vi "New Prop C.vi"(11 "GIC Input":T1={"     Use ?\nOff       On"=[FALSE, TRUE, FALSE, TRUE], "Mode:"=FALSE, "WP Data"="", "Hokuyo Port"="COM7", "Prop  Port"="COM6", "Compass Port"="", "GPS Port"="", "Num of WPs"=0, "WP Lats and Longs"={"WP Lats"=[], "WP Longs"=[]}, "Obst Lats and Longs"={"Obst Lats"=[], "Obst Longs"=[]}, "Parameters"=[], "GPS Data"=[], "Compass"=0.0, "LMS Vector"=[], "Vision Vector"=[], "Direction Cmd"=0.0, "Speed Cmd"=0.0, "WP Vector"=[], "WP Number"=0, "Extra"=0, "SW Map"=[], "Path Cluster"={"Path x node"=[], "Path y node"=[]}} {"Obst Lats and Longs"."Obst Longs" format="%#_8g"; "Obst Lats and Longs"."Obst Lats" format="%#_8g"}) -> ()   [LabVIEW 2014]
uses:
  RLcmd Global.vi
  FRcmd Global.vi
  <vilib>/Instr/_visa.llb/VISA Configure Serial Port (Instr).vi
panel:
  out "Prop VISA Resource Name":refnum<visa-resource-name>
  # "New Prop C"
  # "Input:"
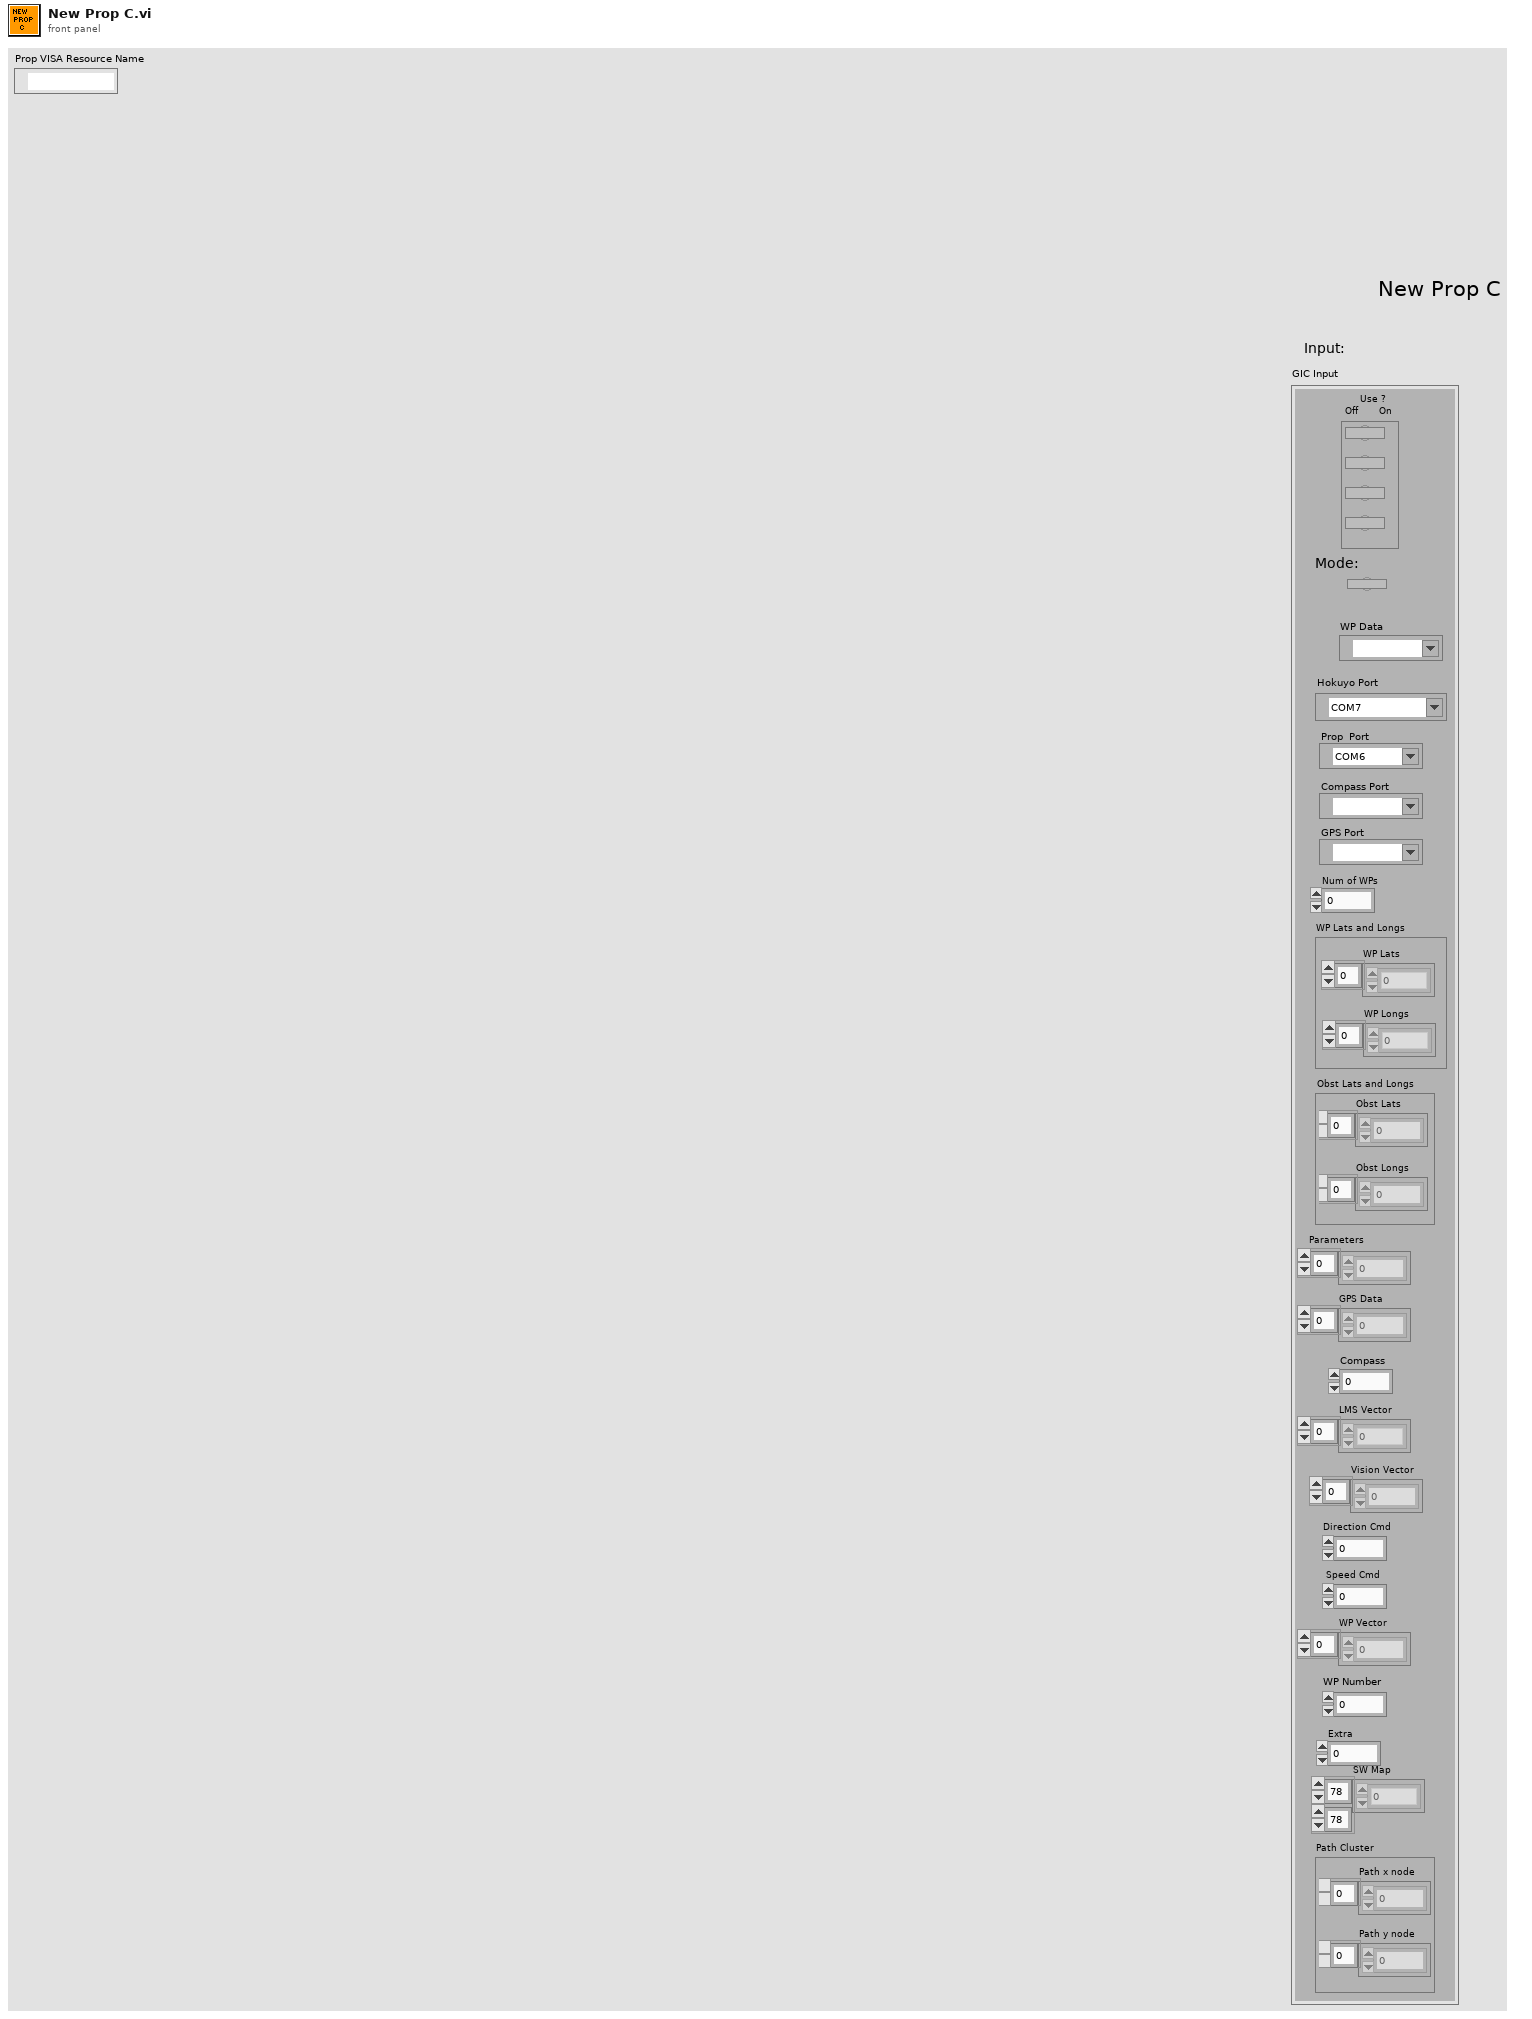
[diagram p1: front panel]
types:
  T1 = cluster{"     Use ?\nOff       On":bool[], "Mode:":bool, "WP Data":refnum<visa-resource-name>, "Hokuyo Port":refnum<visa-resource-name>, "Prop  Port":refnum<visa-resource-name>, "Compass Port":refnum<visa-resource-name>, "GPS Port":refnum<visa-resource-name>, "Num of WPs":i16, "WP Lats and Longs":cluster{"WP Lats":dbl[], "WP Longs":dbl[]}, "Obst Lats and Longs":cluster{"Obst Lats":dbl[], "Obst Longs":dbl[]}, "Parameters":dbl[], "GPS Data":dbl[], "Compass":dbl, "LMS Vector":dbl[], "Vision Vector":dbl[], "Direction Cmd":dbl, "Speed Cmd":dbl, "WP Vector":dbl[], "WP Number":i32, "Extra":i16, "SW Map":i32[][], "Path Cluster":cluster{"Path x node":dbl[], "Path y node":dbl[]}}
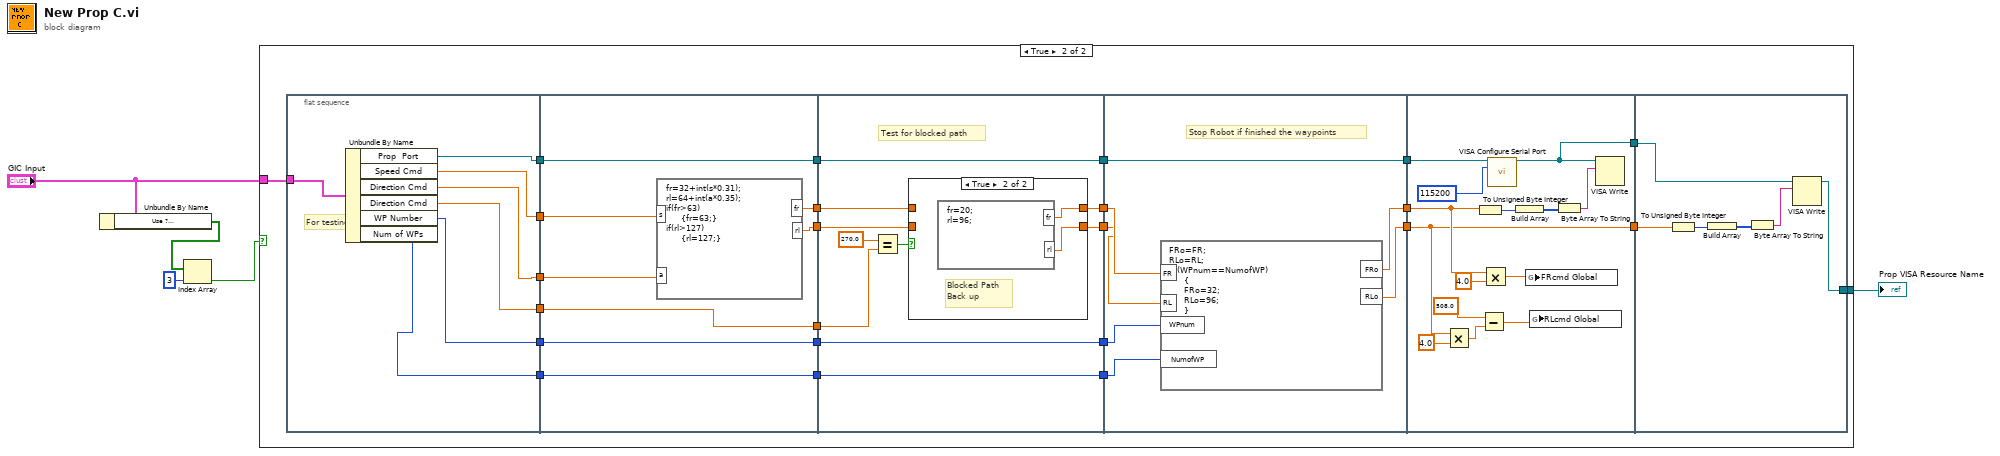
[diagram p0: block diagram]
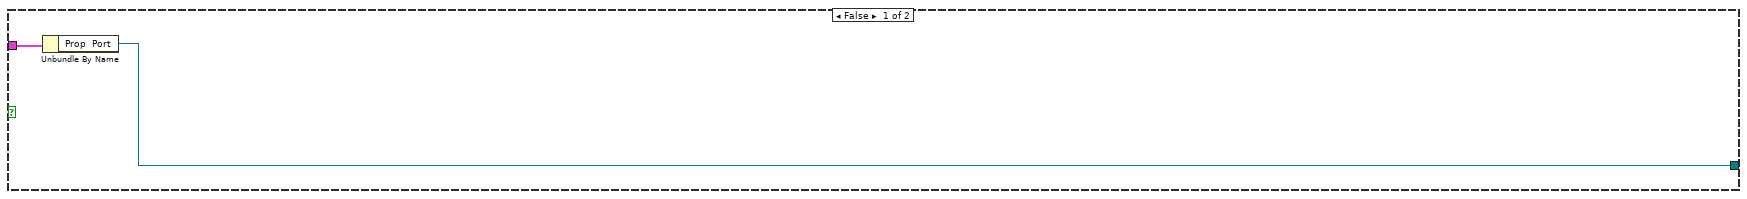
[diagram p2: hidden frame]
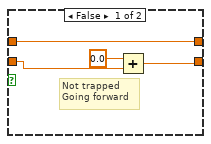
[diagram p3: hidden frame]
diagram:
  n1 = Unbundle By Name("GIC Input") -> ("Use ?\nOff       On"=w5:bool[])
  n2 = Index Array(array=w5, index=3) -> (element=w3:bool)
  n3 = case shown="True" w3 {
    tunnel: "GIC Input" -> [w7 w25]
    tunnel: [w6 w8] -> w2
    frame False {
      n4 = Unbundle By Name(w7) -> ("Prop  Port"=w6:refnum<visa-resource-name>)
    }
    frame True {
      n5 = flat-sequence {
        tunnel: [w38] -> w24
        tunnel: [w37] -> w23
        tunnel: [w36] -> w22
        tunnel: [w35] -> w21
        tunnel: w25 -> [w34]
        tunnel: [w33] -> w12
        tunnel: [w32] -> w9
        tunnel: [w46] -> w31
        tunnel: [w43] -> w30
        tunnel: [w42] -> w29
        tunnel: [w41] -> w28
        tunnel: w21 -> [w41]
        tunnel: w22 -> [w44]
        tunnel: w23 -> [w45]
        tunnel: w24 -> [w46]
        tunnel: [w40] -> w13
        tunnel: w12 -> [w40]
        tunnel: [w39] -> w10
        tunnel: w9 -> [w39]
        tunnel: w31 -> [w56]
        tunnel: [w56] -> w20
        tunnel: w30 -> [w52]
        tunnel: [w51] -> w18
        tunnel: w29 -> [w50]
        tunnel: [w49] -> w16
        tunnel: w28 -> [w53]
        tunnel: [w48] -> w14
        tunnel: w13 -> [w48]
        tunnel: [w47] -> w11
        tunnel: w10 -> [w47]
        tunnel: w20 -> [w69]
        tunnel: [w69] -> w19
        tunnel: w18 -> [w68]
        tunnel: [w66] -> w17
        tunnel: w16 -> [w67]
        tunnel: [w65] -> w15
        tunnel: w14 -> [w64]
        tunnel: w11 -> [w63]
        tunnel: [w79] -> w27
        tunnel: w19 -> [w78]
        tunnel: w17 -> [w77]
        tunnel: [w73] -> w26
        tunnel: w15 -> [w73]
        tunnel: w27 -> [w86]
        tunnel: w26 -> [w85]
        tunnel: [w84] -> w8
        frame #0 {
          # "For testing:"
          n6 = Unbundle By Name(w34) -> ("Prop  Port"=w38:refnum<visa-resource-name>, "Speed Cmd"=w37:dbl, "Direction Cmd"=w36:dbl, "Direction Cmd"=w35:dbl, "WP Number"=w33:i32, "Num of WPs"=w32:i16)
        }
        frame #1 {
          n7 = formula code="fr=32+int(s*0.31);\nrl=64+int(a*0.35);\nif(fr>63)\n     {fr=63;}\nif(rl>127)\n     {rl=127;}"("s"=w45, "a"=w44) -> ("fr"=w43:dbl, "rl"=w42:dbl)
        }
        frame #2 {
          # "Test for blocked path"
          n8 = Equal?(x=270.0, y=w53) -> (x = y?=w55:bool)
          n9 = case shown="True" w55 {
            tunnel: w52 -> [w60 _]
            tunnel: [w60 w62] -> w51
            tunnel: w50 -> [w58 _]
            tunnel: [w59 w61] -> w49
            frame False {
              # "Not trapped\nGoing forward"
              n10 = Add(x=0.0, y=w58) -> (x+y=w59:dbl)
            }
            frame True {
              # "Blocked Path\nBack up"
              n11 = formula code="fr=20;\nrl=96;"() -> ("fr"=w62:dbl, "rl"=w61:dbl)
            }
          }
        }
        frame #3 {
          # "Stop Robot if finished the waypoints"
          n12 = formula code="FRo=FR;\nRLo=RL;\nif (WPnum==NumofWP)\n     {\n     FRo=32;\n     RLo=96;\n     }"("FR"=w68, "RL"=w67, "WPnum"=w64, "NumofWP"=w63) -> ("FRo"=w66:dbl, "RLo"=w65:dbl)
        }
        frame #4 {
          n13 = Multiply(x=w73, y=4.0) -> (x*y=w71:dbl)
          n14 = To Unsigned Byte Integer(number=w77) -> (unsigned 8bit integer=w81:u8)
          n15 = Subtract(x=508.0, y=w71) -> (x-y=w70:dbl)
          n16 = Multiply(x=w77, y=4.0) -> (x*y=w75:dbl)
          n17 = call-poly "VISA Configure Serial Port"("VISA resource name"=w78, "baud rate (9600)"=115200) -> ("VISA resource name out"=w79:refnum<visa-resource-name>)  [unwired: 12 in, 1 out]
          n18 = Build Array(w81) -> (w80:u8[])
          n19 = global write "FRcmd Global.vi" "FRcmd Global"(w75) -> ()
          n20 = global write "RLcmd Global.vi" "RLcmd Global"(w70) -> ()
          n21 = Byte Array To String(unsigned byte array=w80) -> (string=w82:string)
          n22 = VISA Write(VISA resource name=w79, write buffer=w82) -> ()  [unwired: 1 in, 3 out]
        }
        frame #5 {
          n23 = To Unsigned Byte Integer(number=w85) -> (unsigned 8bit integer=w88:u8)
          n24 = Build Array(w88) -> (w89:u8[])
          n25 = Byte Array To String(unsigned byte array=w89) -> (string=w87:string)
          n26 = VISA Write(VISA resource name=w86, write buffer=w87) -> (VISA resource name out=w84:refnum<visa-resource-name>)  [unwired: 1 in, 2 out]
        }
      }
    }
  }
  "Prop VISA Resource Name" <- w2
